vi "Set Date.vi"(5 "Old Specification (T)":bool=TRUE, 6 "Day":i32=1 min=1 max=31 step=1, 7 "Year":i32=7 min=7 max=49 step=1, 8 "error in (no error)":errorcluster, 9 "Month":i32=1 min=1 max=12 step=1, 10 "Address (0)":i32, 11 "VISA resource name":refnum<visa-resource-name>) -> (0 "error out":errorcluster, 3 "VISA resource name out":refnum<visa-resource-name>)   [LabVIEW 2016, in "Environment Chamber.lvlib" / "Climatic Chamber.lvlib"]
doc: "<b>Date setting</B>\n\nChanges the date of the internal calendar."
uses:
  Climatic Chamber.lvlib
panel:
  out "NACK":bool
  out "Error":bool
  out "ACK":bool
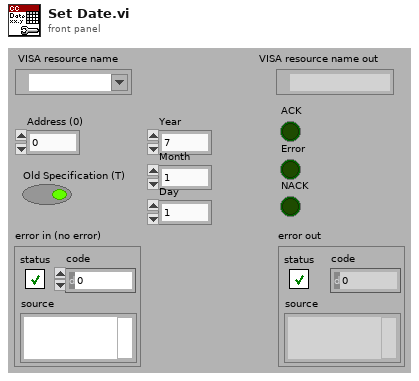
[diagram p1: front panel]
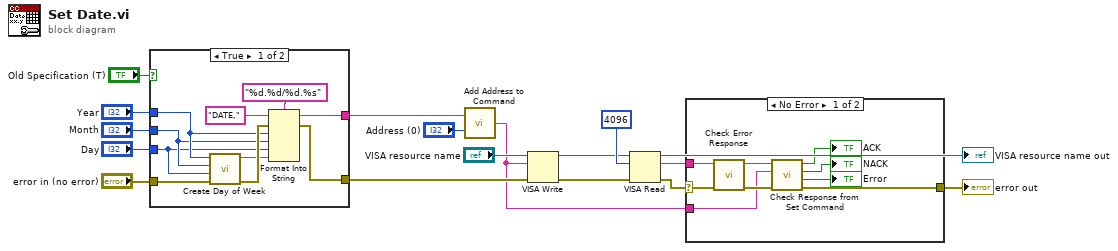
[diagram p0: block diagram]
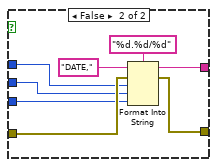
[diagram p2: hidden frame]
diagram:
  n1 = case shown="True" "Old Specification (T)" {
    tunnel: [w24 w32] -> w8
    tunnel: [w23 w31] -> w7
    tunnel: "Year" -> [w21 w30]
    tunnel: "Month" -> [w20 w29]
    tunnel: "Day" -> [w19 w28]
    tunnel: "error in (no error)" -> [w18 w35]
    frame True {
      n2 = call "Create Day of Week.vi"("error in (no error)"=w18, "Day"=w19, "Month"=w20, "Year"=w21) -> ("error out"=w27:errorcluster, "Day of Week"=w22:string)  [unwired: 6 in]
      n3 = Format Into String(format string="%d.%d/%d.%s", initial string="DATE,", error in=w27, w21, w20, w19, w22) -> (resulting string=w24:string, error out=w23:errorcluster)
    }
    frame False {
      n4 = Format Into String(format string="%d.%d/%d", initial string="DATE,", error in=w35, w30, w29, w28) -> (resulting string=w32:string, error out=w31:errorcluster)
    }
  }
  n5 = call "Add Address to Command.vi"("Address (0)"="Address (0)", "Command"=w8) -> ("Command OUT"=w6:string)
  n6 = VISA Write(VISA resource name="VISA resource name", write buffer=w6, error in (no error)=w7) -> (VISA resource name out=w15:refnum<visa-resource-name>, error out=w14:errorcluster)  [unwired: 1 out]
  n7 = VISA Read(VISA resource name=w15, byte count=u32 4096, error in (no error)=w14) -> (VISA resource name out=→"VISA resource name out":refnum<visa-resource-name>, read buffer=w10:string, error out=w11:errorcluster)  [unwired: 1 out]
  n8 = case shown="No Error" w11 {
    selector: w11 -> [w43 w45]
    tunnel: w10 -> [w44 _]
    tunnel: [w39 w45] -> w9
    tunnel: w6 -> [w40 _]
    frame No Error {
      n9 = call "Check Error Response.vi"("error in (no error)"=w43, "read String"=w44) -> ("error out"=w42:errorcluster, "String out"=w41:string)  [unwired: 7 in, 1 out]
      n10 = call "Check Response from Set Command.vi"("error in (no error)"=w42, "Command"=w40, "Response"=w41) -> ("error out"=w39:errorcluster, "Error"=→"Error":bool, "NACK"=→"NACK":bool, "ACK"=→"ACK":bool)  [unwired: 5 in]
    }
    frame Error {
    }
  }
  "error out" <- w9
